vi "Start.vi"(8 "error in":errorcluster, 11 "shared resources in":refnum<class "Shared Resources.lvclass">) -> (0 "error out":errorcluster, 3 "shared resources out":refnum<class "Shared Resources.lvclass">)   [LabVIEW 2020, in "AIM ARINC 429 Engine.lvlib" / "Implementation.lvlib" / "Shared Resources.lvclass"]
uses:
  Shared Resources.lvclass
  Shared Resources.lvclass/Shared Resources.ctl
  <instrlib>/AIM GmbH/ARINC-429/AIM429LV.lvlib
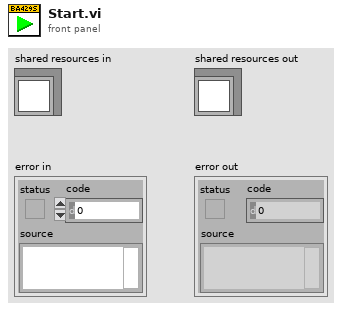
[diagram p1: front panel]
types:
  T1 = typedef "Direction.ctl" = enum16{"Rx", "Tx"}
  T2 = typedef "Transfer Speed.ctl" = enum16{"LO (12.5 kb/s)", "HI (100 kb/s)"}
  T3 = cluster{"channel":u8, "direction":T1, "speed":T2}[]
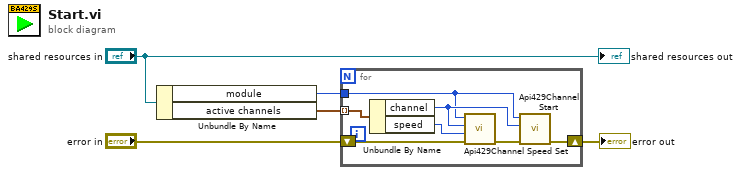
[diagram p0: block diagram]
diagram:
  n1 = Unbundle By Name("shared resources in") -> ("module"=w4:u8, "active channels"=w3:T3)
  n2 = for {
    shift-right: [w12] -> w1
    shift-left: "error in" -> [w7]
    tunnel: w4 -> [w8]
    tunnel: w3 -> [w11] mode=indexing
    n3 = Unbundle By Name(w11) -> ("channel"=w9:u8, "speed"=w10:T2)
    n4 = call <instrlib>:"Api429Channel Speed Set.vi"("error in (no error)"=w7, "speed"=w10, "b_Chn"=w9, "board_handle"=w8) -> ("error out"=w6:errorcluster)  [unwired: 7 in]
    n5 = call <instrlib>:"Api429Channel Start.vi"("error in (no error)"=w6, "channel_id"=w9, "board_handle"=w8) -> ("error out"=w12:errorcluster)  [unwired: 8 in]
  }
  "error out" <- w1
  "shared resources out" <- "shared resources in"
